vi "Remove Section Item By Name.vi"(8 "error in (no error)":errorcluster, 9 "AutoDisposeSubItems(T)":bool=TRUE, 10 "Item Name":string, 11 "Section Reference in":u64 format="%.0x") -> (0 "error out":errorcluster, 3 "Section Reference out":u64 format="%.0x", 4 "success?":bool)   [LabVIEW 2013, in "Hierarchy Framework.lvlib" / "Section.lvclass"]
doc: "Searches for <B>Item Name</B> in the section specified by <B>Section Reference in</B> and, if found, remove and dispose the item from parent <B>Section Reference in</B> ."
uses:
  Section.lvclass
  Generic/Generic.lvclass
  Item/Item.lvclass
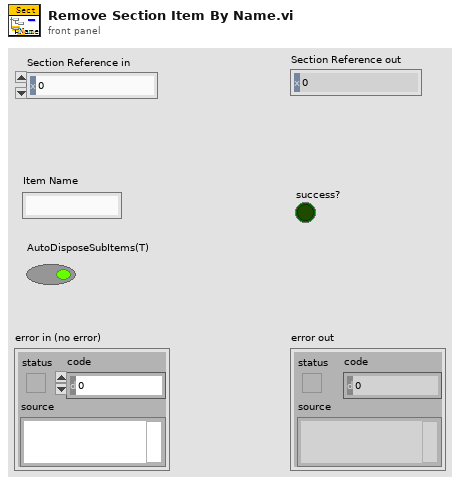
[diagram p1: front panel]
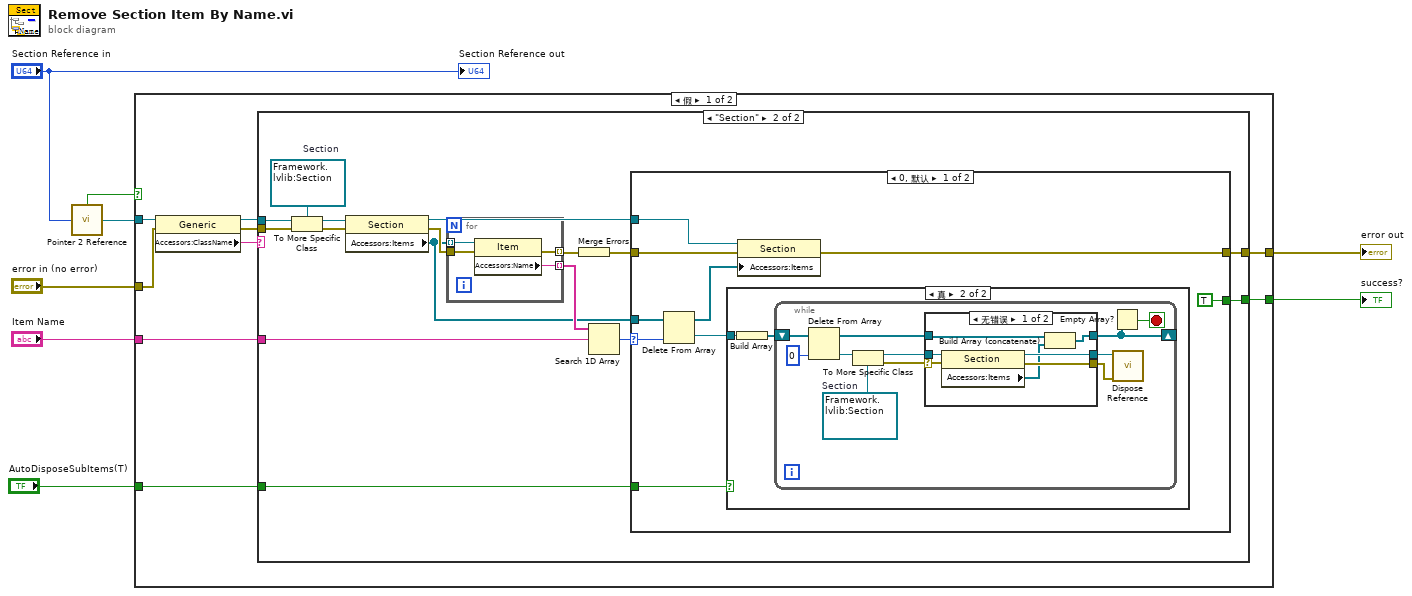
[diagram p0: block diagram]
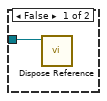
[diagram p3: hidden frame]
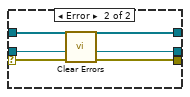
[diagram p4: hidden frame]
diagram:
  n1 = call "Pointer 2 Reference.vi"("Pointer"="Section Reference in") -> ("Not A Refnum?"=w5:bool, "Generic Reference"=w4:refnum<data-value>)
  n2 = case shown="假" w5 {
    tunnel: w4 -> [w16 _]
    tunnel: "error in (no error)" -> [w15 w74]
    tunnel: [w17 w74] -> w7
    tunnel: [w11 _] -> w3
    tunnel: "Item Name" -> [w10 _]
    tunnel: "AutoDisposeSubItems(T)" -> [w9 _]
    frame False {
      n3 = property class="Generic"(reference=w16, error in=w15) -> (reference out=w13:refnum<data-value>, error out=w14:errorcluster, "Accessors:ClassName"=w12:string)
      n4 = case shown="\"Section\"" w12 {
        tunnel: [w18 w20] -> w17
        tunnel: w14 -> [w18 w31]
        tunnel: w13 -> [_ w30]
        tunnel: [_ w23] -> w11
        tunnel: w10 -> [_ w26]
        tunnel: w9 -> [_ w19]
        frame Default {
        }
        frame "Section" {
          w34 = refnum<data-value> refnum  # Section
          n5 = To More Specific Class(target class=w34, reference=w30, error in=w31) -> (specific class reference=w33:refnum<data-value>, error out=w32:errorcluster)
          n6 = property class="Section"(reference=w33, error in=w32) -> (reference out=w22:refnum<data-value>, error out=w28:errorcluster, "Accessors:Items"=w24:refnum<data-value>[])
          n7 = for {
            tunnel: w24 -> [w73] mode=indexing
            tunnel: [w72] -> w27 mode=indexing
            tunnel: w28 -> [w71]
            tunnel: [w70] -> w29 mode=indexing
            n8 = property class="Item"(reference=w73, error in=w71) -> (error out=w70:errorcluster, "Accessors:Name"=w72:string)  [unwired: 1 out]
          }
          n9 = Merge Errors(w29) -> (w21:errorcluster)
          n10 = Search 1D Array(1D array=w27, element=w26) -> (index of element=w25:i32)  [unwired: 1 in]
          n11 = case shown="0, 默认" w25 {
            selector: w25 -> [w43 _]
            tunnel: w24 -> [w42 _]
            tunnel: [TRUE _] -> w23
            tunnel: w22 -> [w40 _]
            tunnel: w21 -> [w38 w69]
            tunnel: [w37 w69] -> w20
            tunnel: w19 -> [w36 _]
            frame 0, Default {
              n12 = Delete From Array(array=w42, index=w43) -> (deleted portion=w35:refnum<data-value>, array with subset deleted=w39:refnum<data-value>[])  [unwired: 1 in]
              n13 = case shown="真" w36 {
                tunnel: w35 -> [w44 w46]
                frame False {
                  n14 = call "Dispose Reference.vi"("Generic Reference"=w44) -> ()  [unwired: 10 in, 1 out]
                }
                frame True {
                  n15 = Build Array(w46) -> (w45:refnum<data-value>[])
                  n16 = while {
                    shift-right: [w48] -> _
                    shift-left: w45 -> [w57]
                    stop <- w47 stop-if-true
                    w54 = refnum<data-value> refnum  # Section
                    n17 = Delete From Array(array=w57, index=0 ("索引")) -> (deleted portion=w55:refnum<data-value>, array with subset deleted=w51:refnum<data-value>[])  [unwired: 1 in]
                    n18 = To More Specific Class(target class=w54, reference=w55) -> (specific class reference=w52:refnum<data-value>, error out=w53:errorcluster)  [unwired: 1 in]
                    n19 = case shown="无错误" w53 {
                      selector: w53 -> [w64 w66]
                      tunnel: w52 -> [w63 w67]
                      tunnel: w51 -> [w62 w68]
                      tunnel: [w61 w68] -> w48
                      tunnel: [w60 w67] -> w50
                      tunnel: [w59 w65] -> w49
                      frame No Error {
                        n20 = property class="Section"(reference=w63, error in=w64) -> (reference out=w60:refnum<data-value>, error out=w59:errorcluster, "Accessors:Items"=w58:refnum<data-value>[])
                        n21 = Build Array (concatenate)(w62, w58) -> (w61:refnum<data-value>[])
                      }
                      frame Error {
                        n22 = call <vilib>:"Clear Errors.vi"("error in (no error)"=w66) -> ("error out"=w65:errorcluster)  [unwired: 6 in]
                      }
                    }
                    n23 = Empty Array?(array=w48) -> (empty?=w47:bool)
                    n24 = call "Dispose Reference.vi"("error in (no error)"=w49, "Generic Reference"=w50) -> ()  [unwired: 9 in, 1 out]
                  }
                }
              }
              n25 = property class="Section"(reference=w40, error in=w38, "Accessors:Items"=w39) -> (error out=w37:errorcluster)  [unwired: 1 out]
            }
            frame -1 {
            }
          }
        }
      }
    }
    frame True {
    }
  }
  "error out" <- w7
  "success?" <- w3
  "Section Reference out" <- "Section Reference in"
